vi "LEBITVacuum.set i attribute.vi"(0 "i ref in":refnum<vi>, 2 "i attribute":T1={"setValuePLC"=[], "nickNames"=[], "setValuePLCServiceID"=[], "monValuePLC"=[], "SetValueServiceID"=[], "MonValueServiceID"=[], "SetValue"=[], "AllPLCValues"=[], "CondSpecial2DArray"=[], "CondSpecialIndex"=[], "ReasonForLocking"="", "ReasonForLockingID"=0, "enableValuePLC"=[], "OverwriteCloseSafetyPLC"=[], "OverwriteOpenSafetyPLC"=[], "OverwriteCloseSafetyPLCServiceID"=[], "OverwriteOpenSafetyPLCServiceID"=[], "MKS Address Array"=[], "MKS MeasurementServiceID"=[], "MKS Measurement"=[], "CRYO Measurement"=[], "CRYO MeasurementServiceID"=[], "Special"=[], "Start Date"="", "MKS VISA resource"="COM13", "CRYO VISA resource"="COM13"}, 5 "error in (no error)":errorcluster) -> (14 "i ref out":refnum<vi>, 19 "error out":errorcluster)   [LabVIEW 2014, in "LEBITVacuum.lvlib"]
doc: "Sets the i attribute data of an object.\n\nLicense Agreement for this software:\n\nCopyright (C)\nGesellschaft für Schwerionenforschung, GSI\nPlanckstr. 1\n64291 Darmstadt\nGermany\n\nContact: D.Beck@gsi.de \n\nThis program is free software; you can redistribute it and/or modify it under the terms of the GNU General Public License as published by the Free Software Foundation; either version 2 of the license, or (at your option) any later version.\n\nThis program is distributed in the hope that it will be useful, but WITHOUT ANY WARRANTY; without even the implied warranty of MERCHANTABILITY or FITNESS FOR A PARTICULAR PURPOSE. See the GNU General License for more details (http://www.gnu.org).\n\nGesellschaft für Schwerionenforschung, GSI\nPlanckstr. 1, 64291 Darmstadt, Germany\nFor all questions and ideas contact: M.Richter@gsi.de, H.Brand@gsi.de or D.Beck@gsi.de.\nLast update: 17-JUN-2004"
uses:
  LEBITVacuum.lvlib
  LEBITVacuum.i attribute.ctl
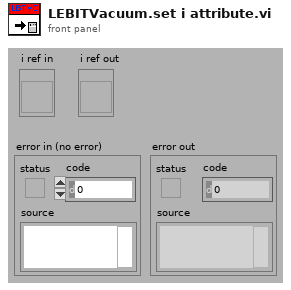
[diagram p1: front panel]
types:
  T1 = typedef "LEBITVacuum.lvlib/LEBITVacuum.i attribute.ctl" = cluster{"setValuePLC":string[], "nickNames":string[], "setValuePLCServiceID":i32[], "monValuePLC":string[], "SetValueServiceID":i32[], "MonValueServiceID":i32[], "SetValue":i16[], "AllPLCValues":string[], "CondSpecial2DArray":string[][], "CondSpecialIndex":i32[], "ReasonForLocking":string, "ReasonForLockingID":i32, "enableValuePLC":string[], "OverwriteCloseSafetyPLC":string[], "OverwriteOpenSafetyPLC":string[], "OverwriteCloseSafetyPLCServiceID":i32[], "OverwriteOpenSafetyPLCServiceID":i32[], "MKS Address Array":i32[][], "MKS MeasurementServiceID":i32[], "MKS Measurement":string[], "CRYO Measurement":string[][], "CRYO MeasurementServiceID":i32[], "Special":string[], "Start Date":string, "MKS VISA resource":refnum<visa-resource-name>, "CRYO VISA resource":refnum<visa-resource-name>}
  T2 = enum16{"SetAttribute", "GetAttribute", "CreateAttribute", "DestroyAttribute", "DestroyAllAtributes"}
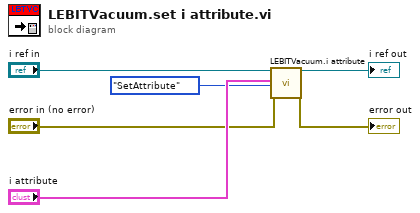
[diagram p0: block diagram]
diagram:
  n1 = call "LEBITVacuum.i attribute.vi"("VI Refnum"="i ref in", "CLASS.i attribute"="i attribute", "Action"=T2."SetAttribute", "error in (no error)"="error in (no error)") -> ("VI Refnum out"=→"i ref out":refnum<vi>, "error out"=→"error out":errorcluster)  [unwired: 13 in, 1 out]
